vi "Start Discovery Service.vi"(8 "error in":errorcluster, 10 "cluster id":string, 11 "key file path":path) -> (0 "error out":errorcluster)   [LabVIEW 2021, in "NI Discovery V1 Client.lvlib"]
doc: "This VI starts the NI Discovery Service."
uses:
  NI Discovery V1 Client.lvlib
  Measurements/Helpers/Error Strings Global Internal.vi
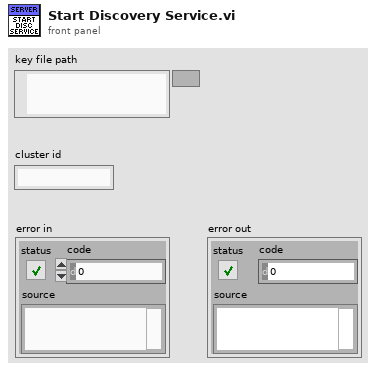
[diagram p1: front panel]
types:
  T1 = enum16{"open", "replace", "create", "open or create", "replace or create", "replace or create with confirmation"}
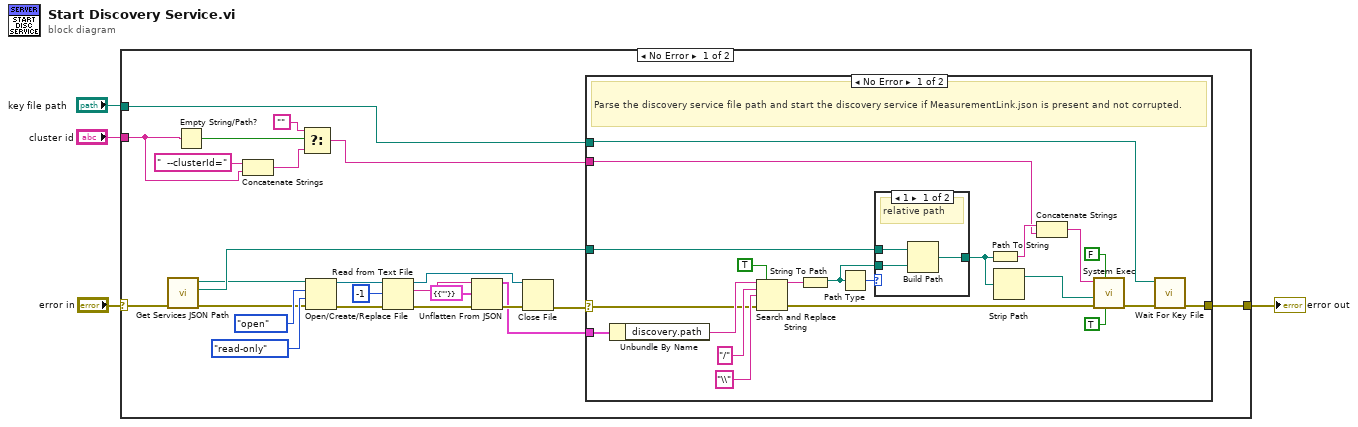
[diagram p0: block diagram]
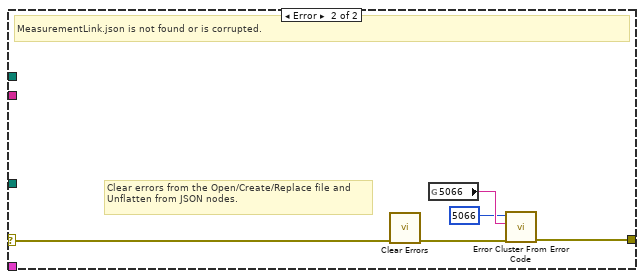
[diagram p3: hidden frame]
diagram:
  n1 = case shown="No Error" "error in" {
    selector: "error in" -> [w8 w59]
    tunnel: [w26 w59] -> w3
    tunnel: "key file path" -> [w25 _]
    tunnel: "cluster id" -> [w13 _]
    frame No Error {
      n2 = call "Get Services JSON Path.vi"("error in (no error)"=w8) -> ("error out"=w5:errorcluster, "services root directory"=w7:path, "services JSON path"=w6:path)  [unwired: 7 in, 1 out]
      n3 = Empty String/Path?(string/path=w13) -> (empty?=w12:bool)
      n4 = Concatenate Strings("  --clusterId=" ("string"), w13) -> (w11:string)
      n5 = Select(t="", s=w12, f=w11) -> (s? t:f=w9:string)
      n6 = Open/Create/Replace File(file path (use dialog)=w6, error in=w5, operation (0:open)=T1."open", access (0:read/write)=enum16{"read/write", "read-only", "write-only"}."read-only") -> (refnum out=w17:refnum<file>, error out=w20:errorcluster)  [unwired: 2 in, 1 out]
      n7 = Read from Text File(file (use dialog)=w17, count=-1, error in=w20) -> (refnum out=w18:refnum<file>, text=w22:string, error out=w24:errorcluster)  [unwired: 1 in, 1 out]
      n8 = Unflatten From JSON(JSON string=w22, type and defaults=cluster{"discovery":cluster{"path":string}} {"discovery"={"path"=""}}, error in (no error)=w24) -> (value=w15:cluster{"discovery":cluster{"path":string}}, error out=w19:errorcluster)  [unwired: 4 in]
      n9 = Close File(refnum=w18, error in=w19) -> (error out=w16:errorcluster)  [unwired: 1 out]
      n10 = case shown="No Error" w16 {
        selector: w16 -> [w33 w58]
        tunnel: [w41 w56] -> w26
        tunnel: w25 -> [w40 _]
        tunnel: w7 -> [w36 _]
        tunnel: w15 -> [w32 _]
        tunnel: w9 -> [w29 _]
        frame No Error {
          # "Parse the discovery service file path and start the discovery service if MeasurementLink.json is present and not corrupted."
          n11 = Unbundle By Name(w32) -> ("discovery.path"=w34:string)
          n12 = Search and Replace String(replace all?=TRUE ("replace all? (F)"), input string=w34, search string="/", replace string="\\" ("replace string (\"\")"), error in=w33) -> (result string=w37:string, error out=w46:errorcluster)  [unwired: 3 in, 2 out]
          n13 = String To Path(string=w37) -> (path=w38:path)
          n14 = Path Type(1:w38) -> (0:w39:i16)
          n15 = case shown="1" w39 {
            tunnel: [w52 w53] -> w35
            tunnel: w36 -> [w51 _]
            tunnel: w38 -> [w50 w53]
            frame 1 {
              # "relative path"
              n16 = Build Path(base path=w51, name or relative path=w50) -> (appended path=w52:path)
            }
            frame Default {
              # "absolute path"
            }
          }
          n17 = Path To String(path=w35) -> (string=w31:string)
          n18 = Strip Path(path=w35) -> (stripped path=w47:path)  [unwired: 1 out]
          n19 = Concatenate Strings(w31, w29) -> (w30:string)
          n20 = call <vilib>:"System Exec.vi"("run minimized? (F)"=TRUE, "wait until completion? (T)"=FALSE, "error in (no error)"=w46, "working directory"=w47, "command line"=w30) -> ("error out"=w43:errorcluster)  [unwired: 3 in, 3 out]
          n21 = call "Wait For Key File.vi"("error in"=w43, "key file path"=w40) -> ("error out"=w41:errorcluster)  [unwired: 9 in]
        }
        frame Error {
          # "Clear errors from the Open/Create/Replace file and Unflatten from JSON nodes."
          # "MeasurementLink.json is not found or is corrupted."
          n22 = call <vilib>:"Clear Errors.vi"("error in (no error)"=w58) -> ("error out"=w57:errorcluster)  [unwired: 5 in, 1 out]
          n23 = global read "Error Strings Global Internal.vi" "5066"() -> (w55:string)
          n24 = call <vilib>:"Error Cluster From Error Code.vi"("error in (no error)"=w57, "error message (\"\")"=w55, "error code (0)"=5066) -> ("error out"=w56:errorcluster)  [unwired: 6 in]
        }
      }
    }
    frame Error {
    }
  }
  "error out" <- w3
